vi "GUI_PW_FrontEnd_Picos.vi"() -> ()   [LabVIEW 2020]
uses:
  Shared/GUI_Template/GUI_master/tcp_new_data_event.ctl
  Shared/GUI_Template/GUI_master/tcp new data cluster.ctl
panel:
  in  "Position.device 11::2":dbl caption="Y" min=-10000.0 max=10000.0
  in  "Position.device 10::2":dbl caption="X" min=-10000.0 max=10000.0
  in  "Position.device 8::2":dbl caption="Y" min=-10000.0 max=10000.0
  in  "Position.device 7::2":dbl caption="X" min=-20000.0 max=20000.0
  in  "Position.device 14::2":dbl caption="Y" min=-1000.0 max=1000.0
  in  "Position.device 13::2":dbl caption="X" min=-1000.0 max=1000.0
  in  "Position.device 5::2":dbl caption="Y" min=-10000.0 max=10000.0
  in  "Position.device 4::2":dbl caption="X" min=-10000.0 max=10000.0
  in  "preamp out step":dbl=10.0 caption="StepSize"
  in  "Move PreAmp Output Up":bool
  in  "Move PreAmp Output Down":bool
  in  "Move PreAmp Output Left":bool
  in  "Move Preamp Output Right":bool
  in  "StepSize\nDogleg":dbl=10.0 caption="StepSize"
  in  "Move Device 11 Neg":bool
  in  "Move Device 11 Pos":bool
  in  "Move Device 10 Pos":bool
  in  "Move Device 10 Neg":bool
  in  "StepSize\nAMP1":dbl=100.0 caption="StepSize"
  in  "Move Device 8 Neg":bool
  in  "Move Device 8 Pos":bool
  in  "Move Device 7 Pos":bool
  in  "Move Device 7 Neg":bool
  in  "StepSize\nPreAmp":dbl=30.0 caption="StepSize"
  in  "Move Device 5 Neg":bool
  in  "Move Device 5 Pos":bool
  in  "Move Device 4 Pos":bool
  in  "Move Device 4 Neg":bool
  in  "StepSize\nXPW":dbl=5.0 caption="StepSize"
  in  "Position.device 2::2":dbl caption="Y" min=-10000.0 max=10000.0
  in  "Move Device 1 Neg":bool
  in  "Move Device 1 Pos":bool
  in  "Move Device 2 Pos":bool
  in  "Move Device 2 Neg":bool
  in  "Position.device 1::2":dbl caption="X" min=-10000.0 max=10000.0
  in  "GUIdevice 2":string="MCD-LT-PicoBooster"
  in  "stop":bool
  out "tcp data event":T1
  out "error IO 2":errorcluster
  # "XPW Input"
  # "Amp 1 Out"
  # "Dogleg"
  # "PreAmp Output"
  # "PreAmp Input"
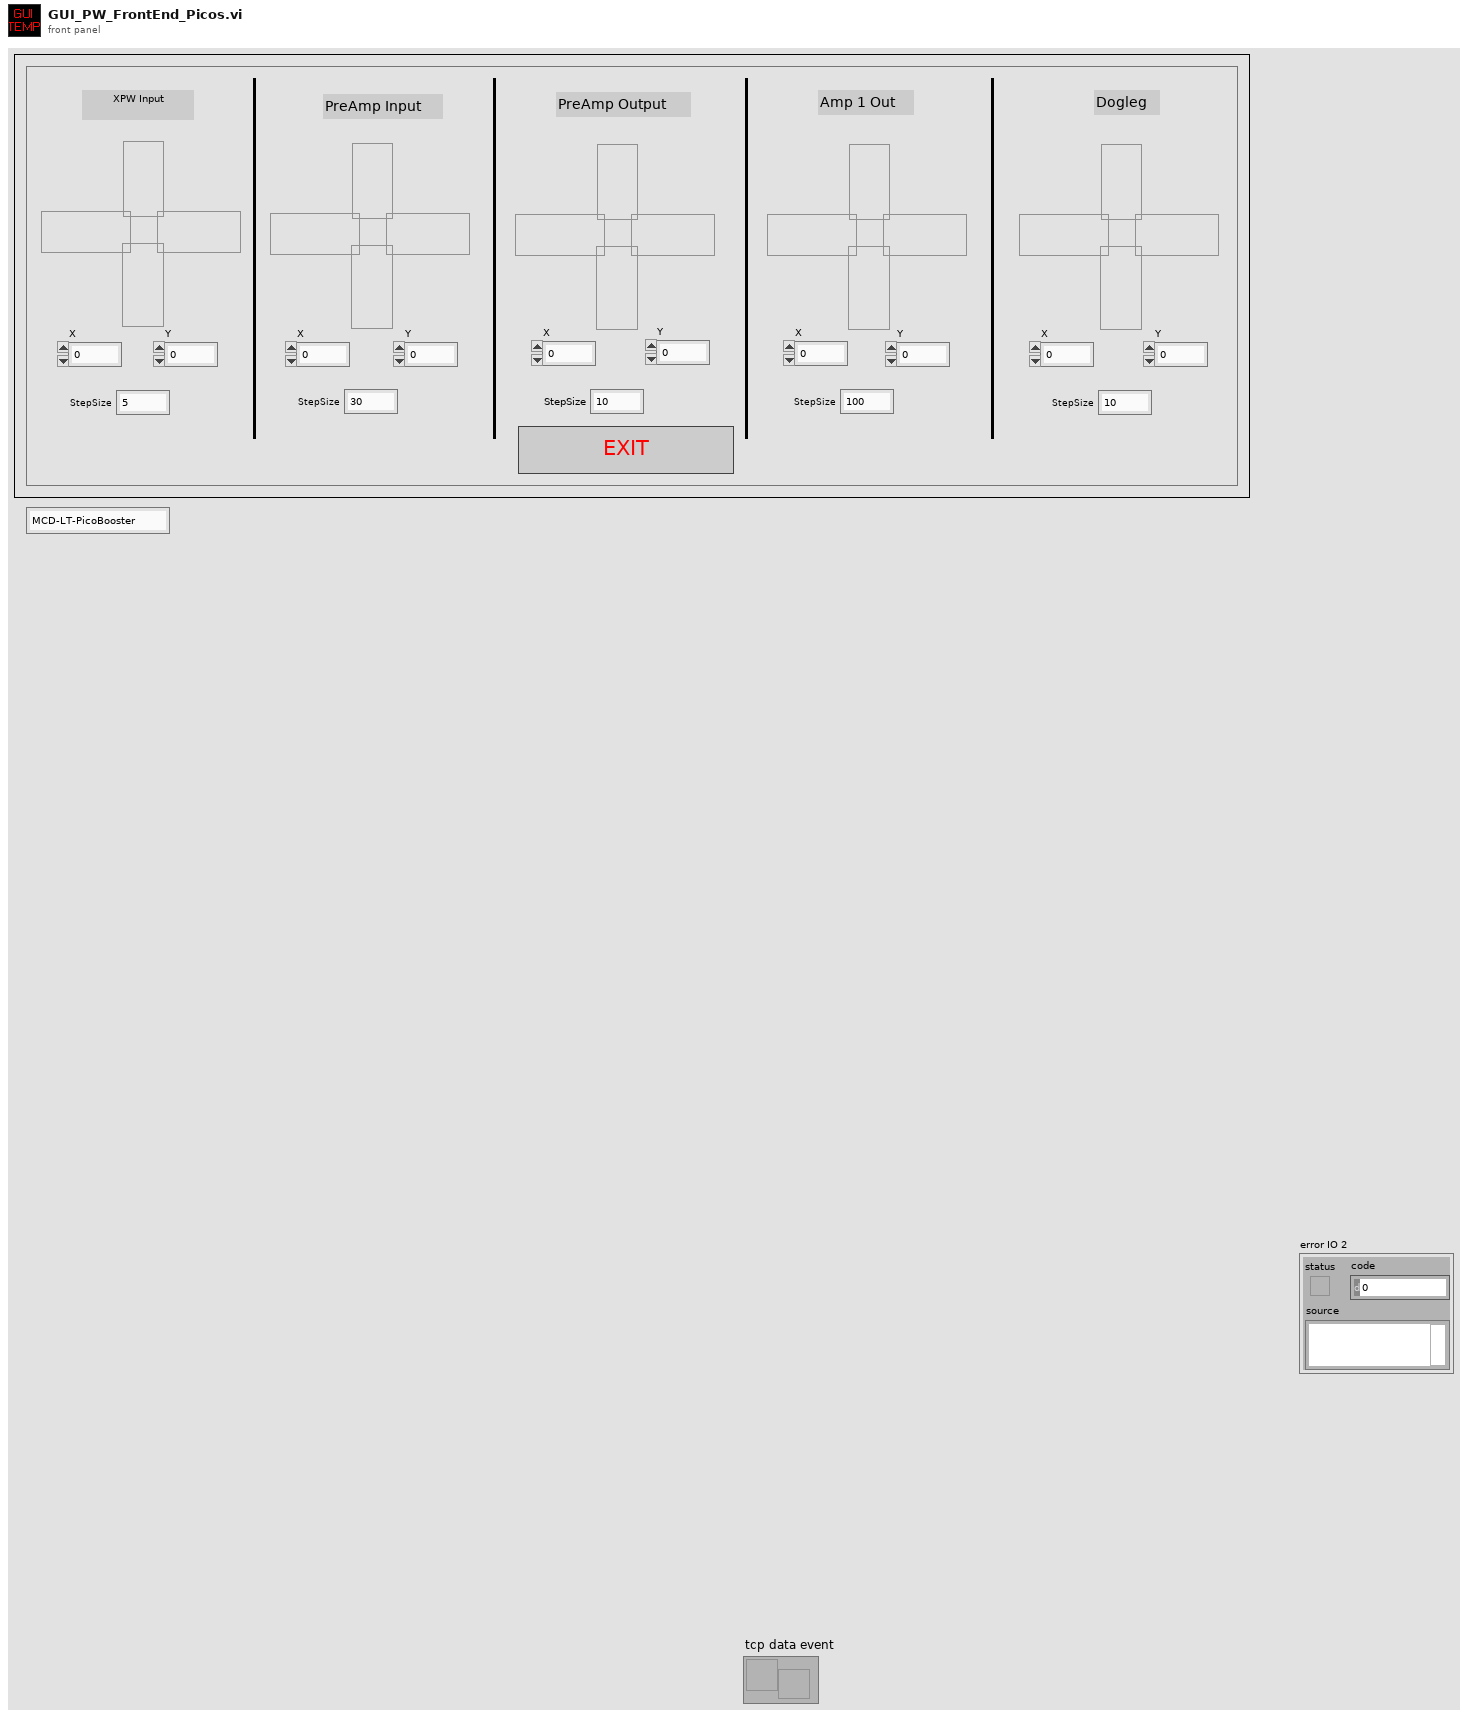
[diagram p1: front panel]
types:
  T1 = typedef "tcp_new_data_event.ctl" = refnum<user-event>
  T2 = typedef "tcp new data cluster.ctl" = cluster{"EventEnum":enum16{"new data", "connection status update"}, "Device name":string}
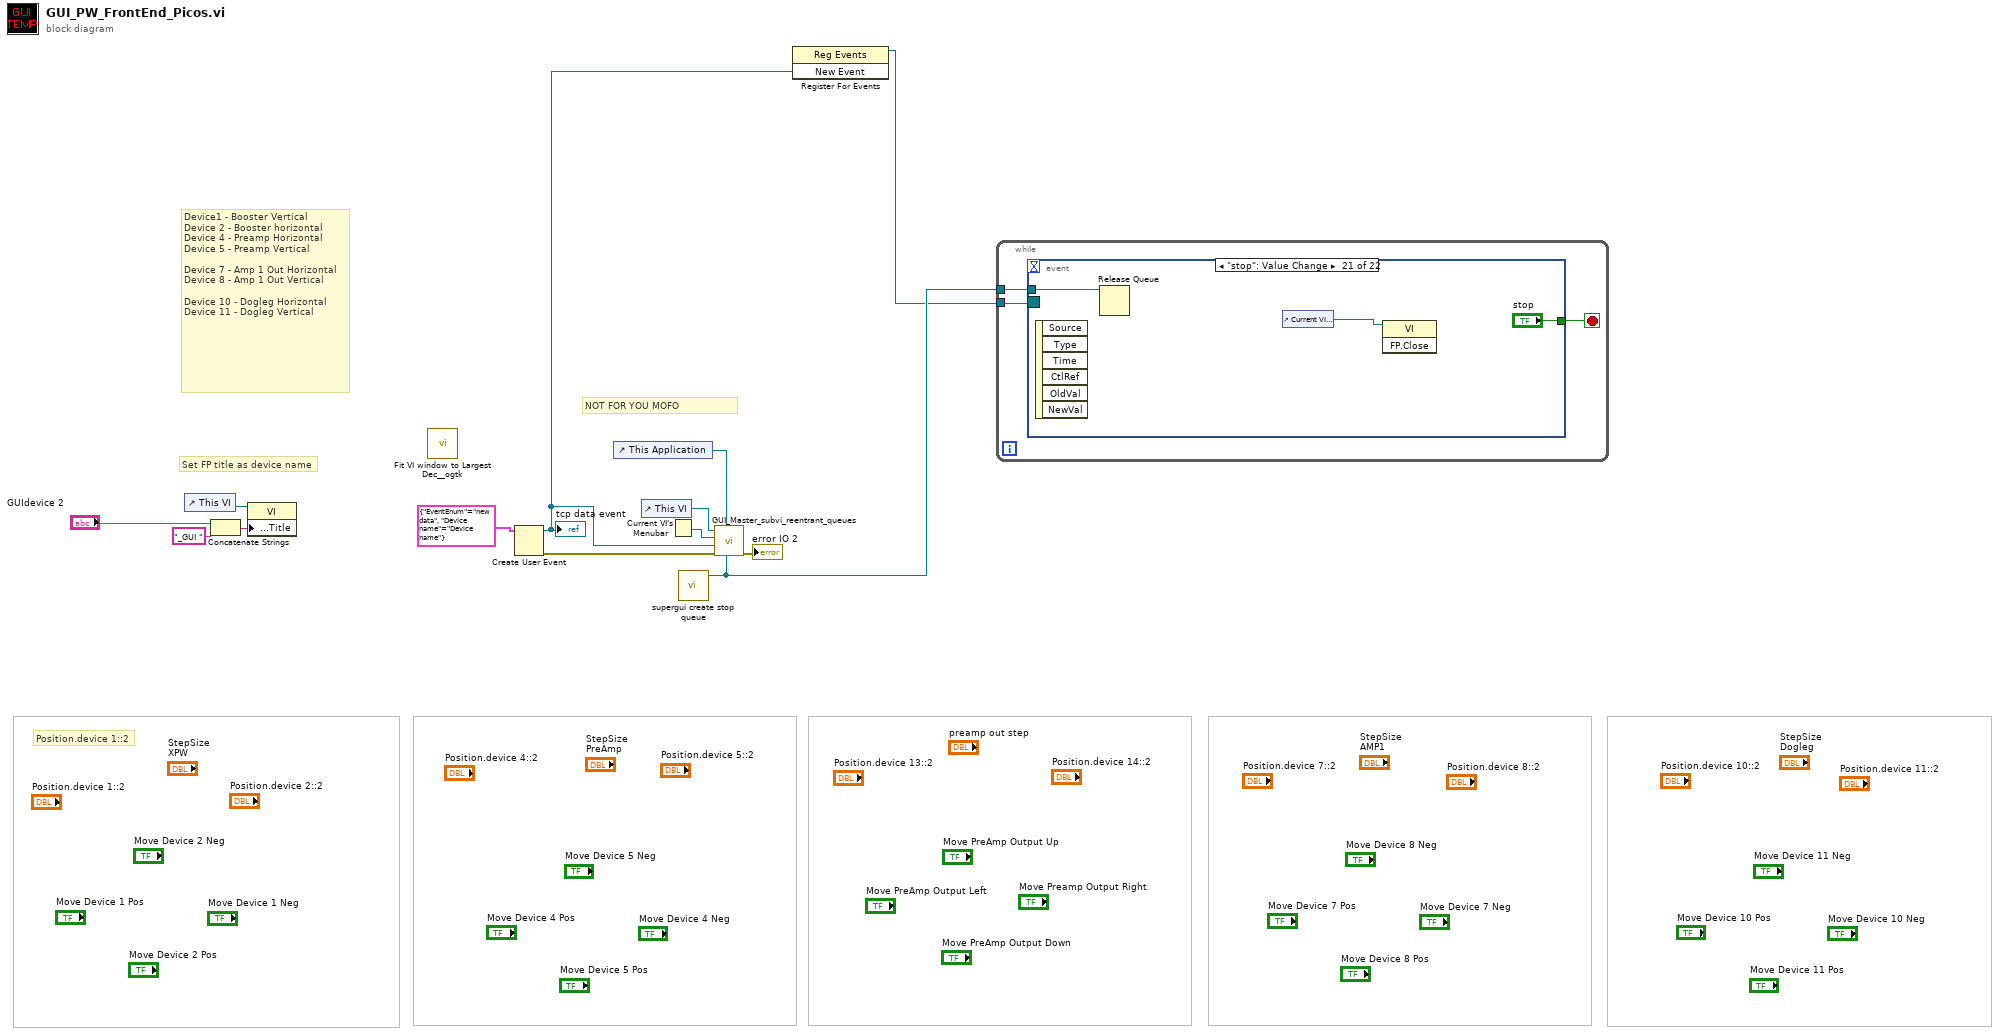
[diagram p0: block diagram]
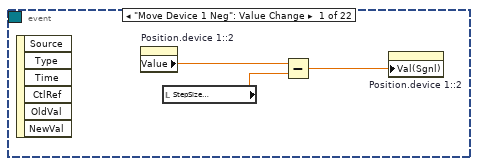
[diagram p2: hidden frame]
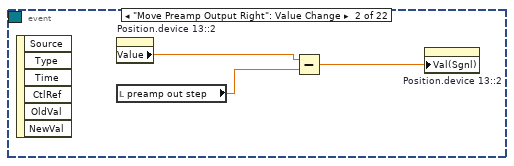
[diagram p3: hidden frame]
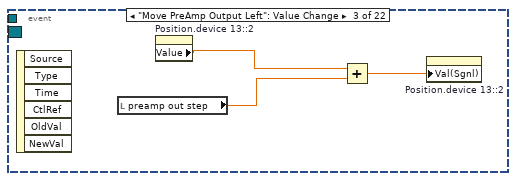
[diagram p4: hidden frame]
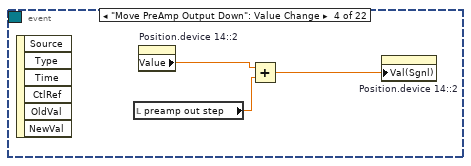
[diagram p5: hidden frame]
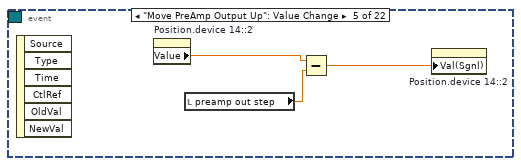
[diagram p6: hidden frame]
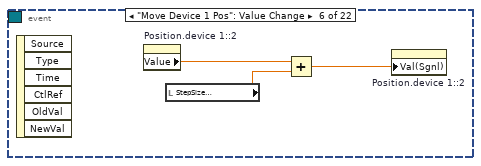
[diagram p7: hidden frame]
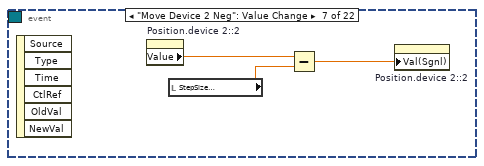
[diagram p8: hidden frame]
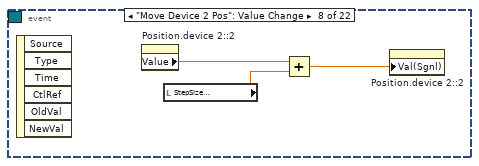
[diagram p9: hidden frame]
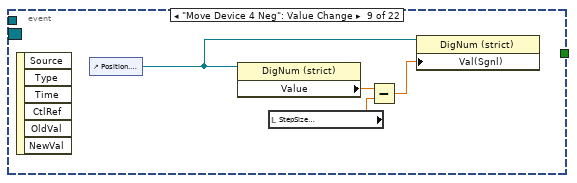
[diagram p10: hidden frame]
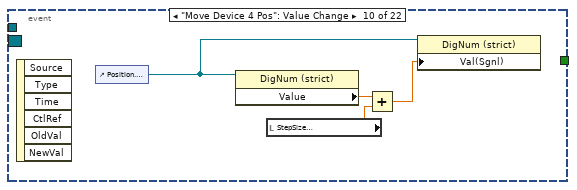
[diagram p11: hidden frame]
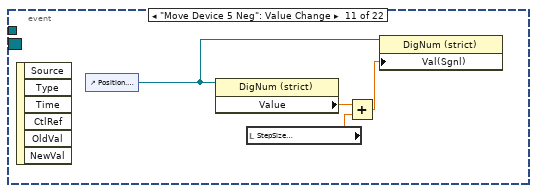
[diagram p12: hidden frame]
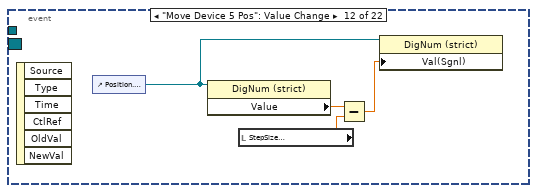
[diagram p13: hidden frame]
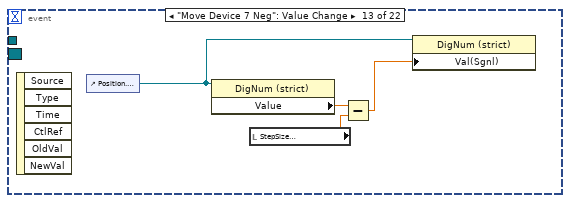
[diagram p14: hidden frame]
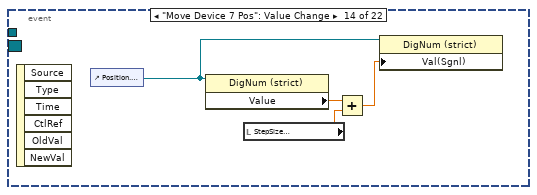
[diagram p15: hidden frame]
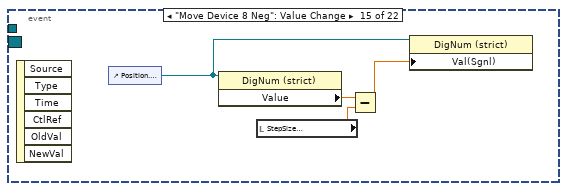
[diagram p16: hidden frame]
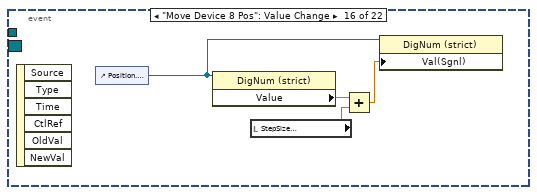
[diagram p17: hidden frame]
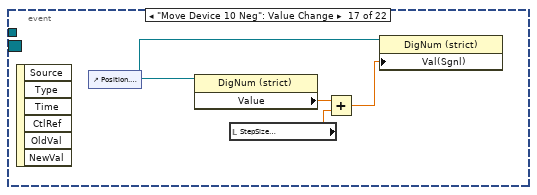
[diagram p18: hidden frame]
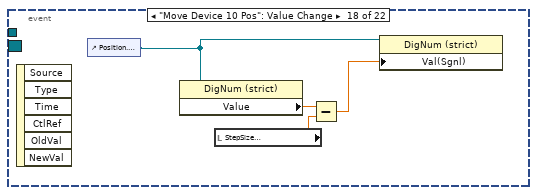
[diagram p19: hidden frame]
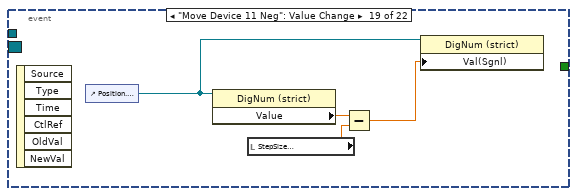
[diagram p20: hidden frame]
diagram:
  # "Position.device 1::2"
  # "Device1 - Booster Vertical\nDevice 2 - Booster horizontal\nDevice 4 - Preamp Horizontal\nDevice 5 - Preamp Vertical\n\nDevice 7 - Amp 1 Out Horizontal\nDevice 8 - Amp 1 Out Vertical\n\nDevice 10 - Dogleg Horizontal\nDevice 11 - Dogleg Vertical"
  # "Set FP title as device name"
  # "NOT FOR YOU MOFO"
  n1 = control-ref of="This VI"() -> (w6:refnum<vi>)
  n2 = Concatenate Strings("GUIdevice 2", "_GUI ") -> (w5:string)
  n3 = property class="VI"(reference=w6, "Front Panel.Title"=w5) -> ()  [unwired: 1 in, 2 out]
  n4 = call <userlib>:"Fit VI window to Largest Dec__ogtk.vi"() -> ()  [unwired: 6 in, 2 out]
  n5 = Create User Event(user event datatype=T2 {"EventEnum"=enum."new data", "Device name"="Device name"} ("New Event")) -> (user event=w8:refnum<user-event>, error out=w9:errorcluster)  [unwired: 1 in]
  "tcp data event" <- w8
  n6 = control-ref of="This Application"() -> (w7:refnum<vi>)
  n7 = control-ref of="This VI"() -> (w12:refnum<vi>)
  n8 = Current VI's Menubar() -> (w11:refnum<k9>)
  n9 = call "supergui create stop queue.vi"() -> ("STOP Queue out"=w2:refnum<queue>)  [unwired: 11 in]
  n10 = call "GUI_Master_subvi_reentrant_queues.vi"("STOP Queue in"=w2, "This Application"=w7, "error in (no error)"=w9, "tcp data event"=w8, "Caller menu reference"=w11, "Caller VI ref"=w12) -> ("error out"=→"error IO 2":errorcluster)  [unwired: 5 in]
  n11 = register-events(w8) -> (reference out=w1:refnum<event-registration>)  [unwired: 2 in, 1 out]
  n12 = while {
    tunnel: w2 -> [w15]
    tunnel: w1 -> [w14]
    stop <- w16 stop-if-true
    n13 = event shown="[20] \"stop\": Value Change" {
      selector: w14 -> [_ _ _ _ _ _ _ _ _ _ _ _ _ _ _ _ _ _ _ _ _ _]
      dyn-events: _ -> [_ _ _ _ _ _ _ _ _ _ _ _ _ _ _ _ _ _ _ _ _ _]
      timeout: _ -> [_ _ _ _ _ _ _ _ _ _ _ _ _ _ _ _ _ _ _ _ _ _]
      tunnel: [_ _ _ _ _ _ _ _ _ _ _ _ _ _ _ _ _ _ _ _ "stop" _] -> w16
      tunnel: w15 -> [_ _ _ _ _ _ _ _ _ _ _ _ _ _ _ _ _ _ _ _ w90 _]
      event "Move Device 1 Neg": Value Change {
        n14 = event-data() -> ()  [unwired: 1 in, 6 out]
        n15 = property on="Position.device 1::2" class="DigNum (strict)"() -> ("Value"=w18:dbl)  [unwired: 2 in, 2 out]
        n16 = local read "StepSize\nXPW"() -> (w19:dbl)
        n17 = Subtract(x=w18, y=w19) -> (x-y=w17:dbl)
        n18 = property on="Position.device 1::2" class="DigNum (strict)"("Val(Sgnl)"=w17) -> ()  [unwired: 2 in, 2 out]
      }
      event "Move Preamp Output Right": Value Change {
        n19 = event-data() -> ()  [unwired: 1 in, 6 out]
        n20 = property on="Position.device 13::2" class="DigNum (strict)"() -> ("Value"=w20:dbl)  [unwired: 2 in, 2 out]
        n21 = local read "preamp out step"() -> (w22:dbl)
        n22 = Subtract(x=w20, y=w22) -> (x-y=w21:dbl)
        n23 = property on="Position.device 13::2" class="DigNum (strict)"("Val(Sgnl)"=w21) -> ()  [unwired: 2 in, 2 out]
      }
      event "Move PreAmp Output Left": Value Change {
        n24 = event-data() -> ()  [unwired: 1 in, 6 out]
        n25 = local read "preamp out step"() -> (w25:dbl)
        n26 = property on="Position.device 13::2" class="DigNum (strict)"() -> ("Value"=w23:dbl)  [unwired: 2 in, 2 out]
        n27 = Add(x=w23, y=w25) -> (x+y=w24:dbl)
        n28 = property on="Position.device 13::2" class="DigNum (strict)"("Val(Sgnl)"=w24) -> ()  [unwired: 2 in, 2 out]
      }
      event "Move PreAmp Output Down": Value Change {
        n29 = event-data() -> ()  [unwired: 1 in, 6 out]
        n30 = local read "preamp out step"() -> (w28:dbl)
        n31 = property on="Position.device 14::2" class="DigNum (strict)"() -> ("Value"=w27:dbl)  [unwired: 2 in, 2 out]
        n32 = Add(x=w27, y=w28) -> (x+y=w26:dbl)
        n33 = property on="Position.device 14::2" class="DigNum (strict)"("Val(Sgnl)"=w26) -> ()  [unwired: 2 in, 2 out]
      }
      event "Move PreAmp Output Up": Value Change {
        n34 = event-data() -> ()  [unwired: 1 in, 6 out]
        n35 = property on="Position.device 14::2" class="DigNum (strict)"() -> ("Value"=w30:dbl)  [unwired: 2 in, 2 out]
        n36 = local read "preamp out step"() -> (w31:dbl)
        n37 = Subtract(x=w30, y=w31) -> (x-y=w29:dbl)
        n38 = property on="Position.device 14::2" class="DigNum (strict)"("Val(Sgnl)"=w29) -> ()  [unwired: 2 in, 2 out]
      }
      event "Move Device 1 Pos": Value Change {
        n39 = event-data() -> ()  [unwired: 1 in, 6 out]
        n40 = property on="Position.device 1::2" class="DigNum (strict)"() -> ("Value"=w33:dbl)  [unwired: 2 in, 2 out]
        n41 = local read "StepSize\nXPW"() -> (w34:dbl)
        n42 = Add(x=w33, y=w34) -> (x+y=w32:dbl)
        n43 = property on="Position.device 1::2" class="DigNum (strict)"("Val(Sgnl)"=w32) -> ()  [unwired: 2 in, 2 out]
      }
      event "Move Device 2 Neg": Value Change {
        n44 = event-data() -> ()  [unwired: 1 in, 6 out]
        n45 = property on="Position.device 2::2" class="DigNum (strict)"() -> ("Value"=w36:dbl)  [unwired: 2 in, 2 out]
        n46 = local read "StepSize\nXPW"() -> (w37:dbl)
        n47 = Subtract(x=w36, y=w37) -> (x-y=w35:dbl)
        n48 = property on="Position.device 2::2" class="DigNum (strict)"("Val(Sgnl)"=w35) -> ()  [unwired: 2 in, 2 out]
      }
      event "Move Device 2 Pos": Value Change {
        n49 = event-data() -> ()  [unwired: 1 in, 6 out]
        n50 = property on="Position.device 2::2" class="DigNum (strict)"() -> ("Value"=w39:dbl)  [unwired: 2 in, 2 out]
        n51 = local read "StepSize\nXPW"() -> (w40:dbl)
        n52 = Add(x=w39, y=w40) -> (x+y=w38:dbl)
        n53 = property on="Position.device 2::2" class="DigNum (strict)"("Val(Sgnl)"=w38) -> ()  [unwired: 2 in, 2 out]
      }
      event "Move Device 4 Neg": Value Change {
        n54 = event-data() -> ()  [unwired: 1 in, 6 out]
        n55 = control-ref of="Position.device 4::2"() -> (w41:refnum<vi>)
        n56 = property on="Property Node" class="DigNum (strict)"(reference=w41) -> ("Value"=w43:dbl)  [unwired: 1 in, 2 out]
        n57 = local read "StepSize\nPreAmp"() -> (w44:dbl)
        n58 = Subtract(x=w43, y=w44) -> (x-y=w42:dbl)
        n59 = property on="Property Node" class="DigNum (strict)"(reference=w41, "Val(Sgnl)"=w42) -> ()  [unwired: 1 in, 2 out]
      }
      event "Move Device 4 Pos": Value Change {
        n60 = event-data() -> ()  [unwired: 1 in, 6 out]
        n61 = control-ref of="Position.device 4::2"() -> (w45:refnum<vi>)
        n62 = property on="Property Node" class="DigNum (strict)"(reference=w45) -> ("Value"=w47:dbl)  [unwired: 1 in, 2 out]
        n63 = local read "StepSize\nPreAmp"() -> (w48:dbl)
        n64 = Add(x=w47, y=w48) -> (x+y=w46:dbl)
        n65 = property on="Property Node" class="DigNum (strict)"(reference=w45, "Val(Sgnl)"=w46) -> ()  [unwired: 1 in, 2 out]
      }
      event "Move Device 5 Neg": Value Change {
        n66 = event-data() -> ()  [unwired: 1 in, 6 out]
        n67 = control-ref of="Position.device 5::2"() -> (w49:refnum<vi>)
        n68 = property on="Property Node" class="DigNum (strict)"(reference=w49) -> ("Value"=w51:dbl)  [unwired: 1 in, 2 out]
        n69 = local read "StepSize\nPreAmp"() -> (w52:dbl)
        n70 = Add(x=w51, y=w52) -> (x+y=w50:dbl)
        n71 = property on="Property Node" class="DigNum (strict)"(reference=w49, "Val(Sgnl)"=w50) -> ()  [unwired: 1 in, 2 out]
      }
      event "Move Device 5 Pos": Value Change {
        n72 = event-data() -> ()  [unwired: 1 in, 6 out]
        n73 = control-ref of="Position.device 5::2"() -> (w53:refnum<vi>)
        n74 = property on="Property Node" class="DigNum (strict)"(reference=w53) -> ("Value"=w55:dbl)  [unwired: 1 in, 2 out]
        n75 = local read "StepSize\nPreAmp"() -> (w56:dbl)
        n76 = Subtract(x=w55, y=w56) -> (x-y=w54:dbl)
        n77 = property on="Property Node" class="DigNum (strict)"(reference=w53, "Val(Sgnl)"=w54) -> ()  [unwired: 1 in, 2 out]
      }
      event "Move Device 7 Neg": Value Change {
        n78 = event-data() -> ()  [unwired: 1 in, 6 out]
        n79 = control-ref of="Position.device 7::2"() -> (w57:refnum<vi>)
        n80 = property on="Property Node" class="DigNum (strict)"(reference=w57) -> ("Value"=w59:dbl)  [unwired: 1 in, 2 out]
        n81 = local read "StepSize\nAMP1"() -> (w60:dbl)
        n82 = Subtract(x=w59, y=w60) -> (x-y=w58:dbl)
        n83 = property on="Property Node" class="DigNum (strict)"(reference=w57, "Val(Sgnl)"=w58) -> ()  [unwired: 1 in, 2 out]
      }
      event "Move Device 7 Pos": Value Change {
        n84 = event-data() -> ()  [unwired: 1 in, 6 out]
        n85 = control-ref of="Position.device 7::2"() -> (w61:refnum<vi>)
        n86 = property on="Property Node" class="DigNum (strict)"(reference=w61) -> ("Value"=w63:dbl)  [unwired: 1 in, 2 out]
        n87 = local read "StepSize\nAMP1"() -> (w64:dbl)
        n88 = Add(x=w63, y=w64) -> (x+y=w62:dbl)
        n89 = property on="Property Node" class="DigNum (strict)"(reference=w61, "Val(Sgnl)"=w62) -> ()  [unwired: 1 in, 2 out]
      }
      event "Move Device 8 Neg": Value Change {
        n90 = event-data() -> ()  [unwired: 1 in, 6 out]
        n91 = control-ref of="Position.device 8::2"() -> (w65:refnum<vi>)
        n92 = property on="Property Node" class="DigNum (strict)"(reference=w65) -> ("Value"=w67:dbl)  [unwired: 1 in, 2 out]
        n93 = local read "StepSize\nAMP1"() -> (w68:dbl)
        n94 = Subtract(x=w67, y=w68) -> (x-y=w66:dbl)
        n95 = property on="Property Node" class="DigNum (strict)"(reference=w65, "Val(Sgnl)"=w66) -> ()  [unwired: 1 in, 2 out]
      }
      event "Move Device 8 Pos": Value Change {
        n96 = event-data() -> ()  [unwired: 1 in, 6 out]
        n97 = control-ref of="Position.device 8::2"() -> (w69:refnum<vi>)
        n98 = property on="Property Node" class="DigNum (strict)"(reference=w69) -> ("Value"=w71:dbl)  [unwired: 1 in, 2 out]
        n99 = local read "StepSize\nAMP1"() -> (w72:dbl)
        n100 = Add(x=w71, y=w72) -> (x+y=w70:dbl)
        n101 = property on="Property Node" class="DigNum (strict)"(reference=w69, "Val(Sgnl)"=w70) -> ()  [unwired: 1 in, 2 out]
      }
      event "Move Device 10 Neg": Value Change {
        n102 = event-data() -> ()  [unwired: 1 in, 6 out]
        n103 = control-ref of="Position.device 10::2"() -> (w73:refnum<vi>)
        n104 = property on="Property Node" class="DigNum (strict)"(reference=w73) -> ("Value"=w75:dbl)  [unwired: 1 in, 2 out]
        n105 = local read "StepSize\nDogleg"() -> (w76:dbl)
        n106 = Add(x=w75, y=w76) -> (x+y=w74:dbl)
        n107 = property on="Property Node" class="DigNum (strict)"(reference=w73, "Val(Sgnl)"=w74) -> ()  [unwired: 1 in, 2 out]
      }
      event "Move Device 10 Pos": Value Change {
        n108 = event-data() -> ()  [unwired: 1 in, 6 out]
        n109 = control-ref of="Position.device 10::2"() -> (w77:refnum<vi>)
        n110 = property on="Property Node" class="DigNum (strict)"(reference=w77) -> ("Value"=w79:dbl)  [unwired: 1 in, 2 out]
        n111 = local read "StepSize\nDogleg"() -> (w80:dbl)
        n112 = Subtract(x=w79, y=w80) -> (x-y=w78:dbl)
        n113 = property on="Property Node" class="DigNum (strict)"(reference=w77, "Val(Sgnl)"=w78) -> ()  [unwired: 1 in, 2 out]
      }
      event "Move Device 11 Neg": Value Change {
        n114 = event-data() -> ()  [unwired: 1 in, 6 out]
        n115 = control-ref of="Position.device 11::2"() -> (w81:refnum<vi>)
        n116 = property on="Property Node" class="DigNum (strict)"(reference=w81) -> ("Value"=w83:dbl)  [unwired: 1 in, 2 out]
        n117 = local read "StepSize\nDogleg"() -> (w84:dbl)
        n118 = Subtract(x=w83, y=w84) -> (x-y=w82:dbl)
        n119 = property on="Property Node" class="DigNum (strict)"(reference=w81, "Val(Sgnl)"=w82) -> ()  [unwired: 1 in, 2 out]
      }
      event "Move Device 11 Pos": Value Change {
        n120 = event-data() -> ()  [unwired: 1 in, 6 out]
        n121 = control-ref of="Position.device 11::2"() -> (w85:refnum<vi>)
        n122 = property on="Property Node" class="DigNum (strict)"(reference=w85) -> ("Value"=w87:dbl)  [unwired: 1 in, 2 out]
        n123 = local read "StepSize\nDogleg"() -> (w88:dbl)
        n124 = Add(x=w87, y=w88) -> (x+y=w86:dbl)
        n125 = property on="Property Node" class="DigNum (strict)"(reference=w85, "Val(Sgnl)"=w86) -> ()  [unwired: 1 in, 2 out]
      }
      event "stop": Value Change {
        n126 = event-data() -> ()  [unwired: 1 in, 6 out]
        n127 = Release Queue(queue=w90) -> ()  [unwired: 2 in, 3 out]
        n128 = control-ref of="Current VI Reference"() -> (w89:refnum<vi>)
        n129 = invoke class="VI" method="FP.Close"(reference=w89) -> ()  [unwired: 2 in, 3 out]
      }
      event Timeout {
        n130 = event-data() -> ()  [unwired: 1 in, 3 out]
      }
    }
  }
